vi "connect to error stream.vi"(6 "message scheduler":refnum<class "message scheduler.lvclass">, 9 "Queues":T1, 11 "comms in":T2) -> (3 "comms out":T2)   [LabVIEW 2018]
uses:
  type defs/comms loop data.ctl
  ICL-LabVIEW_General/Incident logger/Incident logger.lvclass
  <vilib>/Modbus/master/Modbus Master.lvclass
  type defs/Queues.ctl
  ICL-LabVIEW_General/Message Scheduler/message scheduler.lvclass
  ICL-LabVIEW_General/Message Scheduler/generic message queue/standard message queue/standard message.lvclass
  C:/GitHub/ICL-LabVIEW_General/Message Scheduler/generic message queue/generic message.lvclass
  supporting VIs/polymorphic VIs/enqueue for comms.vi
  supporting VIs/polymorphic VIs/enqueue for message handler.vi
  ICL-LabVIEW_General/Message Scheduler/scheduled message/scheduled message.lvclass
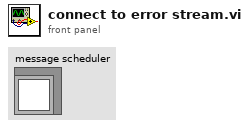
[diagram p1: front panel]
types:
  T1 = typedef "Queues.ctl" = cluster{"messageHandler":refnum<queue>, "comms":refnum<queue>, "dataStream":refnum<queue>, "dataProcessor":refnum<queue>, "fileIO":refnum<queue>, "userInterface":refnum<queue>, "errors":refnum<queue>, "customCompressor":refnum<queue>}
  T2 = typedef "comms loop data.ctl" = cluster{"params":cluster{"commandStream":cluster{"reader name":string, "writer name":string, "stream buffer size":i32}, "errorStream":cluster{"reader name":string, "writer name":string, "stream buffer size":i32}, "RT IP address":string, "pulserControllerIP":string}, "vars":cluster{"commandStream":refnum<k21>, "Incident logger":refnum<class "Incident logger.lvclass">, "check error scheduled message":u32, "errorStream":refnum<k21>, "watchdogScheduleID":u32, "pulsator":cluster{"pulser connection":refnum<class "Modbus Master.lvclass">, "pulserConnected":bool, "pulsatorScheduleID":u32, "pulserRunning":bool, "pulsatorRetries":u8}}}
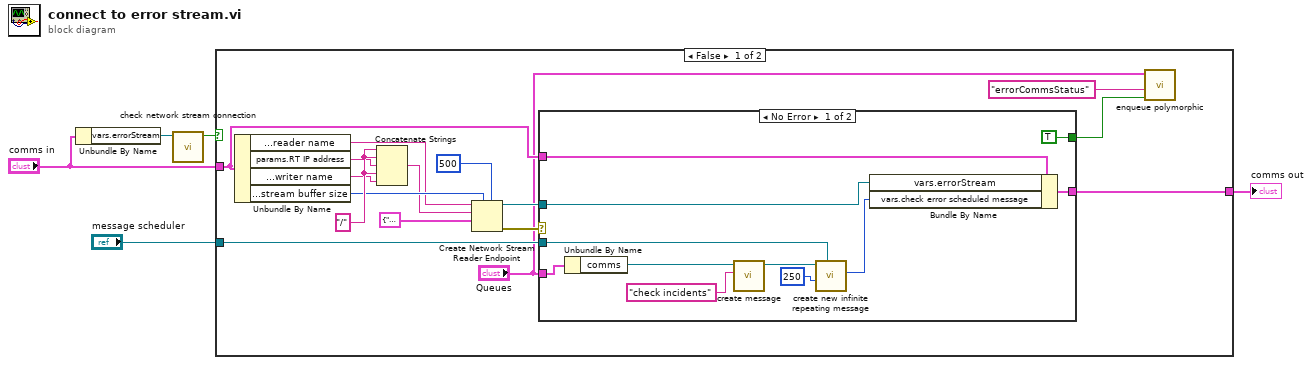
[diagram p0: block diagram]
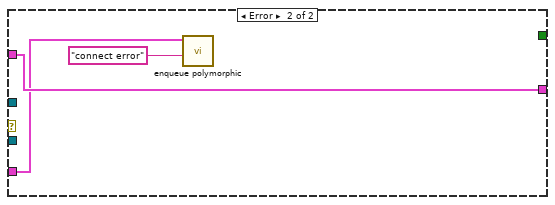
[diagram p2: hidden frame]
diagram:
  n1 = Unbundle By Name("comms in") -> ("vars.errorStream"=w2:refnum<k21>)
  n2 = call "check network stream connection.vi"("stream ref"=w2) -> ("Connected"=w1:bool)  [unwired: 10 in]
  n3 = case shown="False" w1 {
    tunnel: "comms in" -> [w19 w36]
    tunnel: [w20 w36] -> w4
    tunnel: "message scheduler" -> [w10 _]
    frame False {
      w21 = "/" ("string")
      n4 = Unbundle By Name(w19) -> ("params.errorStream.reader name"=w15:string, "params.RT IP address"=w14:string, "params.errorStream.writer name"=w13:string, "params.errorStream.stream buffer size"=w16:i32)
      n5 = Concatenate Strings(w21, w21, w14, w21, w13) -> (w12:string)
      n6 = Create Network Stream Reader Endpoint(5:500 ("timeout in ms (-1)"), 7:w16, 9:cluster{"message":string, "data":variant} {"message"="", "data"=variant}, 10:w12, 11:w15) -> (0:w18:errorcluster, 3:w11:refnum<k21>)  [unwired: 2 in]
      n7 = case shown="No Error" w18 {
        tunnel: w19 -> [w30 w35]
        tunnel: [w32 w35] -> w20
        tunnel: w11 -> [w31 _]
        tunnel: w10 -> [w25 _]
        tunnel: "Queues" -> [w29 w33]
        tunnel: [TRUE _] -> w8
        frame No Error {
          n8 = Unbundle By Name(w29) -> ("comms"=w28:refnum<queue>)
          n9 = call "create message.vi"("message"="check incidents", "queue ref"=w28) -> ("standard message out"=w26:refnum<class "standard message.lvclass">)  [unwired: 8 in, 1 out]
          n10 = call "create new infinite repeating message.vi"("message scheduler"=w25, "ms delay"=u32 250, "message"=w26) -> ("schedule ID"=w23:u32)  [unwired: 7 in, 1 out]
          n11 = Bundle By Name(cluster=w30, "vars.errorStream"=w31, "vars.check error scheduled message"=w23) -> (w32:T2)
        }
        frame Error {
          n12 = call-poly "enqueue polymorphic.vi"("message"="connect error", "Queues"=w33) -> ()  [unwired: 9 in, 1 out]
        }
      }
      n13 = call-poly "enqueue polymorphic.vi"("data"=w8, "message"="errorCommsStatus", "Queues"="Queues") -> ()  [unwired: 8 in, 1 out]
    }
    frame True {
    }
  }
  "comms out" <- w4
